vi "Examples - Basic ITC-SA.vi"(5 "Loop Controls":T7={"Heater"=FALSE, "Gas"=FALSE, "PID"=FALSE, "P (K)"=10.0, "I (mins)"=1.0, "D (mins)"=0.0, "Gas set point (%)"=0.0, "Htr Set V (V)"=0.0, "Target T(K)"=0.0, "Htr Set P (W)"=0.0, "Ramp Mode"=FALSE, "Target Rate(K/min)"=0.0, "Ramp End T(K)"=0.0} {"Ramp End T(K)" min=0.0 max=1000.0 step=0.0001 format="%_5g"; "Target Rate(K/min)" min=0.0 max=1000.0 step=0.0001 format="%_5g"; "Htr Set P (W)" min=0.0 max=80.0 step=0.0001 format="%_5g"; "Target T(K)" min=0.0 max=1000.0 step=0.0001 format="%_5g"; "Htr Set V (V)" min=0.0 max=40.0 step=0.0001 format="%_4g"; "Gas set point (%)" min=0.0 max=100.0 step=0.01 format="%_3g"; "D (mins)" min=0.0 max=300.0 step=0.001 format="%_4g"; "I (mins)" min=0.001 max=200.0 step=0.001 format="%_4g"; "P (K)" min=0.1 max=1000.0 step=0.001 format="%.3g"}, 11 "error in (no error)":errorcluster) -> (6 "Temperature (K)":dbl format="%_5g", 8 "Heater V (V)":dbl format="%_4g", 10 "Heater P (W)":dbl format="%_5g", 14 "Gas Open (%)":dbl(slide) scale=0.0..100.0, 15 "error out":errorcluster)   [LabVIEW 2013]
uses:
  <instrlib>/Mercury iXX/Public/Controls/Comms Transport Layer.ctl
  <instrlib>/Mercury iXX/Public/Controls/Serial Settings.ctl
  <instrlib>/Mercury iXX/Public/Controls/ISOBus Address.ctl
  <instrlib>/Mercury iXX/Public/Libraries/Control Loop/Controls/PID cluster.ctl
  <instrlib>/Mercury iXX/Public/Libraries/System/Open/Open System.vi
  <instrlib>/Mercury iXX/Public/Libraries/System/Read/Catalogue (Read).vi
  <instrlib>/Mercury iXX/Public/Libraries/Temperature/Open/Open Temperature Device.vi
  <instrlib>/Mercury iXX/Public/Libraries/Temperature/Configuration/Read/Nickname (Read).vi
  <instrlib>/Mercury iXX/Public/Libraries/Control Loop/Configuration/Read/Auto PID Filename (Read).vi
  <instrlib>/Mercury iXX/Public/Libraries/Control Loop/Configuration/Read/Heater Association (Read).vi
  <instrlib>/Mercury iXX/Public/Libraries/Heater/Open/Open Heater Device.vi
  <instrlib>/Mercury iXX/Public/Libraries/Heater/Configuration/Read/Voltage Limit (Read).vi
  <instrlib>/Mercury iXX/Public/Libraries/Control Loop/Configuration/Read/Auxiliary Association (Read).vi
  <instrlib>/Mercury iXX/Public/Libraries/Auxiliary/Open/Open Auxiliary Device.vi
  <instrlib>/Mercury iXX/Public/Libraries/Heater/Signals/Read/Voltage (Read).vi
  <instrlib>/Mercury iXX/Public/Libraries/Heater/Signals/Read/Power (Read).vi
  <instrlib>/Mercury iXX/Public/Libraries/Temperature/Signals/Read/Temperature (Read).vi
  <instrlib>/Mercury iXX/Public/Libraries/Control Loop/Configuration/Read/PID (Read).vi
  <instrlib>/Mercury iXX/Public/Libraries/Control Loop/Configuration/Read/PID Auto (Read).vi
  <instrlib>/Mercury iXX/Public/Libraries/Control Loop/Configuration/Read/Heater Auto (Read).vi
  <instrlib>/Mercury iXX/Public/Libraries/Control Loop/Configuration/Read/Flow Auto (Read).vi
  <instrlib>/Mercury iXX/Public/Libraries/Control Loop/Configuration/Read/Percentage Heat (Read).vi
  <instrlib>/Mercury iXX/Public/Libraries/Control Loop/Configuration/Set/Temperature Setpoint (Set).vi
  <instrlib>/Mercury iXX/Public/Libraries/Auxiliary/Signals/Read/Percent Open (Read).vi
  <instrlib>/Mercury iXX/Public/Libraries/Control Loop/Configuration/Set/Heater Auto (Set).vi
  <instrlib>/Mercury iXX/Public/Libraries/Control Loop/Configuration/Set/Flow Auto (Set).vi
  <instrlib>/Mercury iXX/Public/Libraries/Control Loop/Configuration/Set/PID Auto (Set).vi
  <instrlib>/Mercury iXX/Public/Libraries/Control Loop/Configuration/Set/D Value (Set).vi
  <instrlib>/Mercury iXX/Public/Libraries/Control Loop/Configuration/Set/I Value (Set).vi
  <instrlib>/Mercury iXX/Public/Libraries/Control Loop/Configuration/Set/P Value (Set).vi
  <instrlib>/Mercury iXX/Public/Libraries/Heater/Configuration/Read/Nominal Resistance (Read).vi
  <instrlib>/Mercury iXX/Public/Libraries/Control Loop/Configuration/Set/Percentage Heat (Set).vi
  <instrlib>/Mercury iXX/Public/Libraries/Control Loop/Configuration/Set/Percentage Flow (Set).vi
  <instrlib>/Mercury iXX/Mercury iXX.lvlib
  <instrlib>/Mercury iXX/Public/Libraries/System.lvlib
  <instrlib>/Mercury iXX/Public/Libraries/Temperature.lvlib
  <instrlib>/Mercury iXX/Public/Libraries/Heater.lvlib
  <instrlib>/Mercury iXX/Public/Libraries/Auxiliary.lvlib
  <instrlib>/Mercury iXX/Public/Libraries/Control Loop.lvlib
panel:
  in  "stop":bool
  in  "Tab Control":T1(tab)=enum."Configuration"
  in  "Connections":T5={"VISA resource name"="", "IP Address"="", "Comms Layer"=enum."Ethernet TCP/IP", "Serial Configuration"={"Baud Rate"=9600, "Parity"=0, "Data Bits"=8, "Stop Bits"=10, "Flow Control"=0}, "Clear Previous Connections (False)"=FALSE, "ID Query (True)"=TRUE, "ISOBUS address"=-1} {"Serial Configuration"."Flow Control" items=["None", "XON/XOFF", "RTS/CTS", "XON/XOFF & RTS/CTS", "DTR/DSR", "XON/XOFF & DTR/DSR"]; "Serial Configuration"."Stop Bits" items=["1.0"=10, "2.0"=20]; "Serial Configuration"."Data Bits" items=["7"=7, "8"=8]; "Serial Configuration"."Parity" items=["None", "Odd", "Even"]; "Serial Configuration"."Baud Rate" items=["300"=300, "600"=600, "1200"=1200, "2400"=2400, "4800"=4800, "9600"=9600, "19200"=19200]}
  out "# of Instruments":i32
  out "Serial Number(s)":string[](array[string])
  out "S/W Version(s)":string[](array[string])
  out "Devices":string[](array[string])
  in  "Connect":bool
  in  "Ramp mode: Interval between target updates (s)":dbl=10.0 min=0.25 max=60.0 step=0.25
  in  "Loop Dev Id's":T6={"Temperure Dev Id"="MB1.T1:TEMP", "Heater Dev Id"="MB0.H1:HTR", "Gas Cntl Dev Id"="DB4.G1:AUX", "Loop Has Gas Cntl?"=FALSE}
  out "Voltage Limit":dbl format="%.2g"
  out "Heater UID":string
  out "Gas Cntl UID":string
  out "Control Sensor":string
  out "Auto PID Filename:":string
  out "GAS":bool
  out "HEAT":bool
  out "Heater (%)":dbl(slide) scale=0.0..100.0
  out "String":string
  out "PID":T8 {"D" min=0.0 max=299.9 step=0.1 format="%#.1f"; "I" min=0.0 max=199.9 step=0.1 format="%#.1f"; "P" min=0.0 max=199.9 step=0.1 format="%#.1f"}
  out "PID":bool
  in  "Log file":string="C:\\temp\\test.lvm"
  out "Strip Chart":T9(graph)
  in  "Log?":bool
  # "Loop Mode\nAuto?"
  # "MercuryiTC-VI"
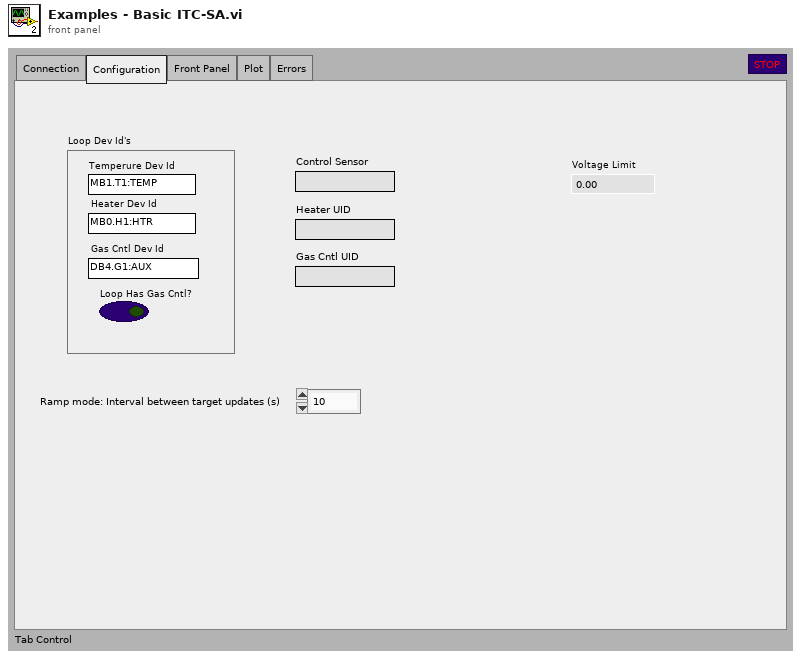
[diagram p1: front panel]
types:
  T1 = enum32{"Connection", "Configuration", "Front Panel", "Plot", "Errors"}
  T2 = typedef "Mercury iXX.lvlib/Comms Transport Layer.ctl" = enum16{"Ethernet TCP/IP", "USB", "ISOBus - RS-232", "GPIB"}
  T3 = typedef "Mercury iXX.lvlib/Serial Settings.ctl" = cluster{"Baud Rate":u32, "Parity":u16, "Data Bits":u16, "Stop Bits":u16, "Flow Control":u16}
  T4 = typedef "Mercury iXX.lvlib/ISOBus Address.ctl" = i32
  T5 = cluster{"VISA resource name":refnum<visa-resource-name>, "IP Address":string, "Comms Layer":T2, "Serial Configuration":T3, "Clear Previous Connections (False)":bool, "ID Query (True)":bool, "ISOBUS address":T4}
  T6 = cluster{"Temperure Dev Id":string, "Heater Dev Id":string, "Gas Cntl Dev Id":string, "Loop Has Gas Cntl?":bool}
  T7 = cluster{"Heater":bool, "Gas":bool, "PID":bool, "P (K)":dbl, "I (mins)":dbl, "D (mins)":dbl, "Gas set point (%)":dbl, "Htr Set V (V)":dbl, "Target T(K)":dbl, "Htr Set P (W)":dbl, "Ramp Mode":bool, "Target Rate(K/min)":dbl, "Ramp End T(K)":dbl}
  T8 = typedef "Mercury iXX.lvlib/Control Loop.lvlib/PID cluster.ctl" = cluster{"P":dbl, "I":dbl, "D":dbl}
  T9 = cluster{"Temperature":dbl, "Percentage Heat":dbl, "% Open":dbl}
  T10 = typedef "Mercury iXX.lvlib/Mercury Reference.ctl" = cluster{"Comms":refnum<visa-resource-name>, "Device ID":string[], "Comms Layer":T2, "Command":string, "Query reference":T11}
  T11 = typedef "Mercury iXX.lvlib/Query Dynamic Reference.ctl" = refnum<vi>
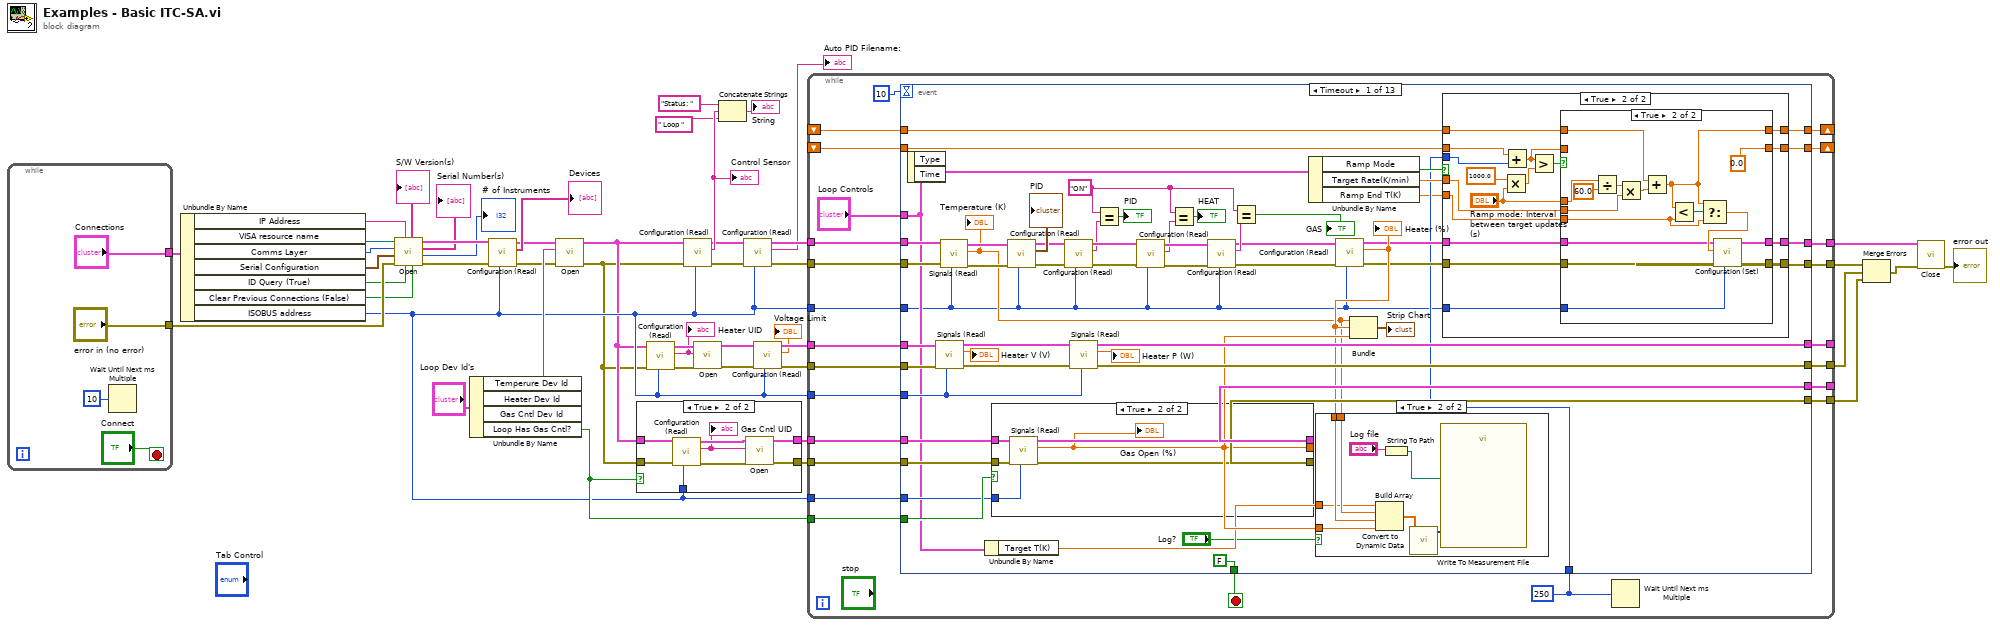
[diagram p0: block diagram]
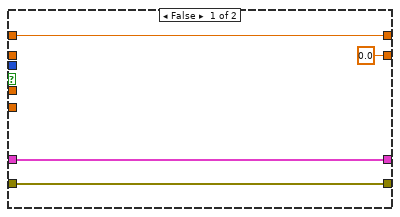
[diagram p3: hidden frame]
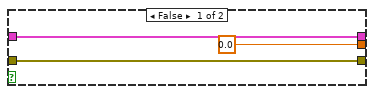
[diagram p6: hidden frame]
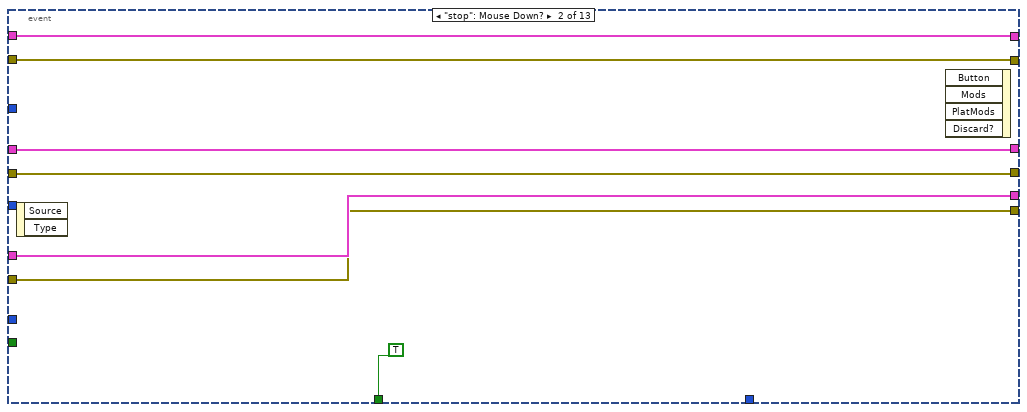
[diagram p7: hidden frame]
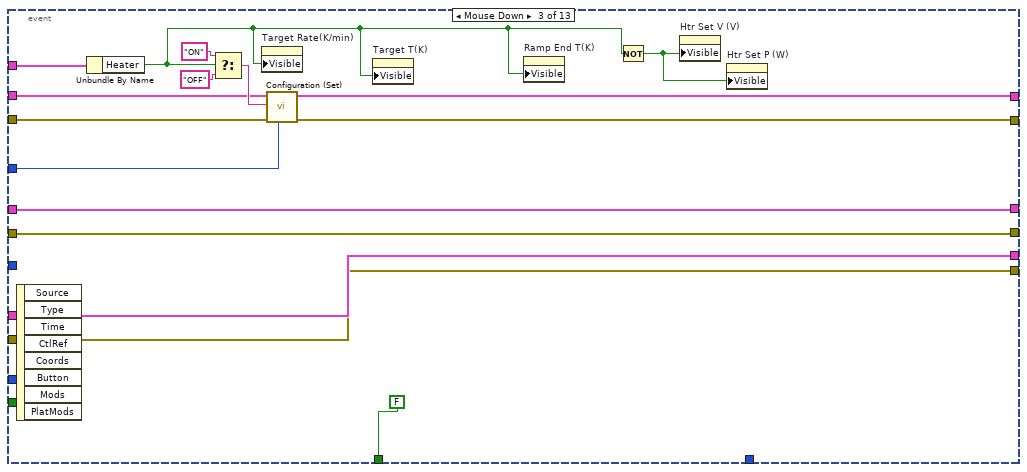
[diagram p8: hidden frame]
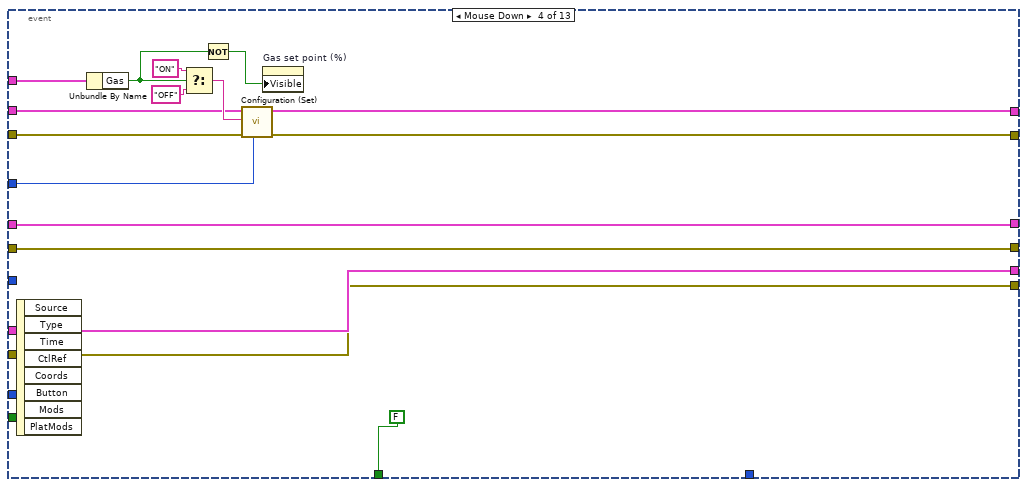
[diagram p9: hidden frame]
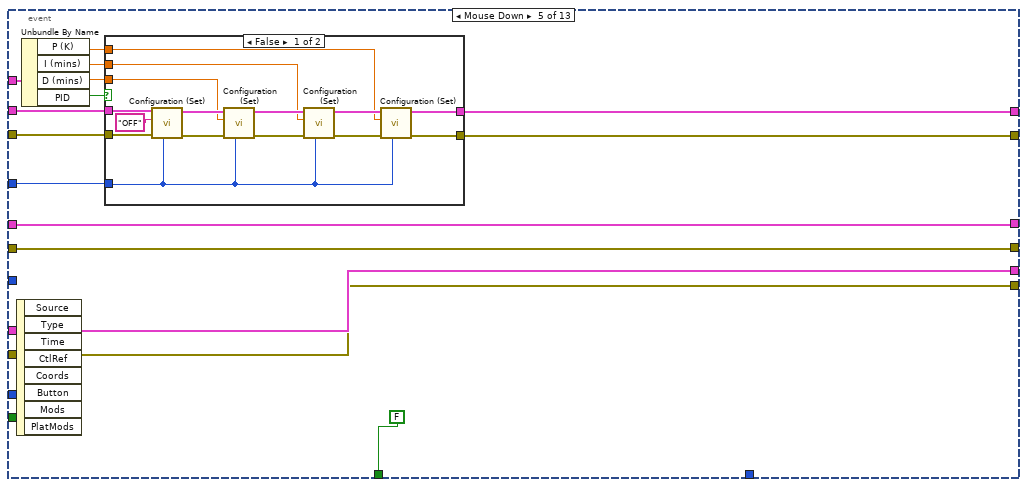
[diagram p10: hidden frame]
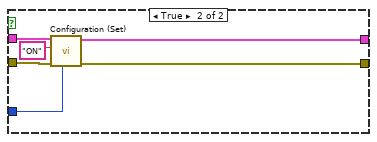
[diagram p11: hidden frame]
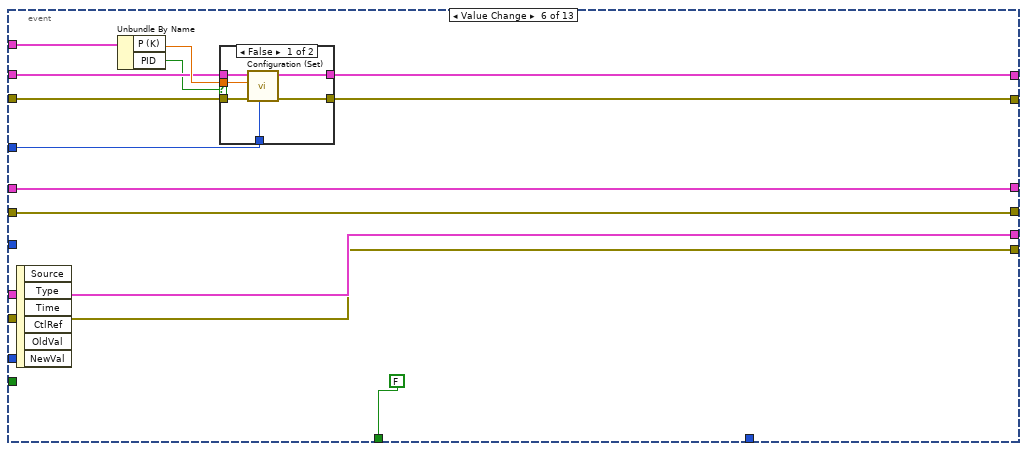
[diagram p12: hidden frame]
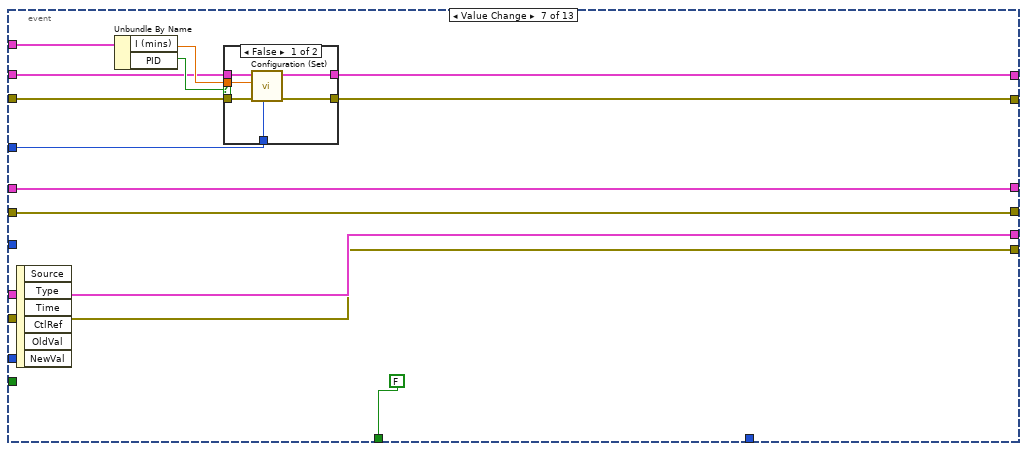
[diagram p14: hidden frame]
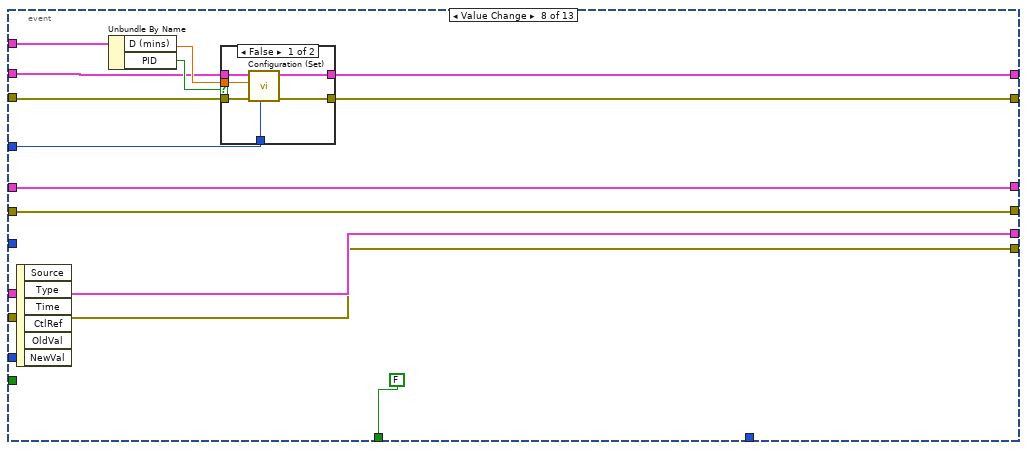
[diagram p16: hidden frame]
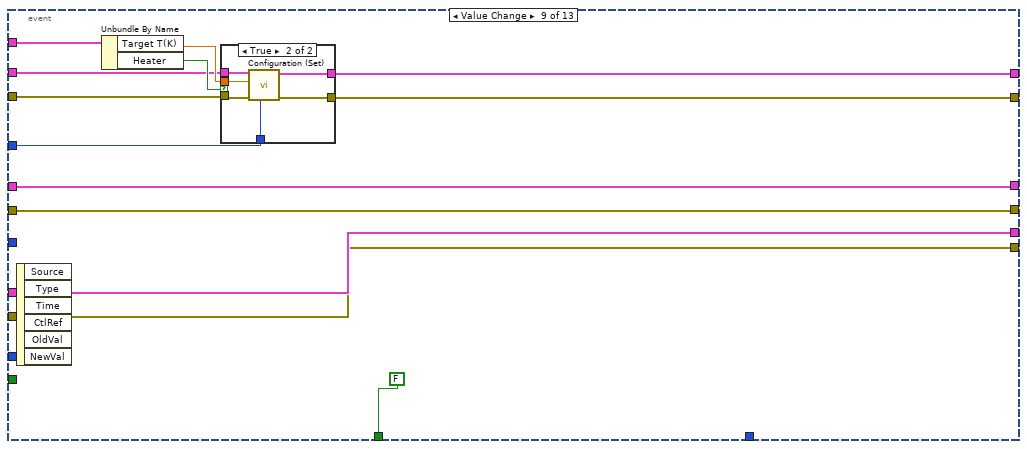
[diagram p18: hidden frame]
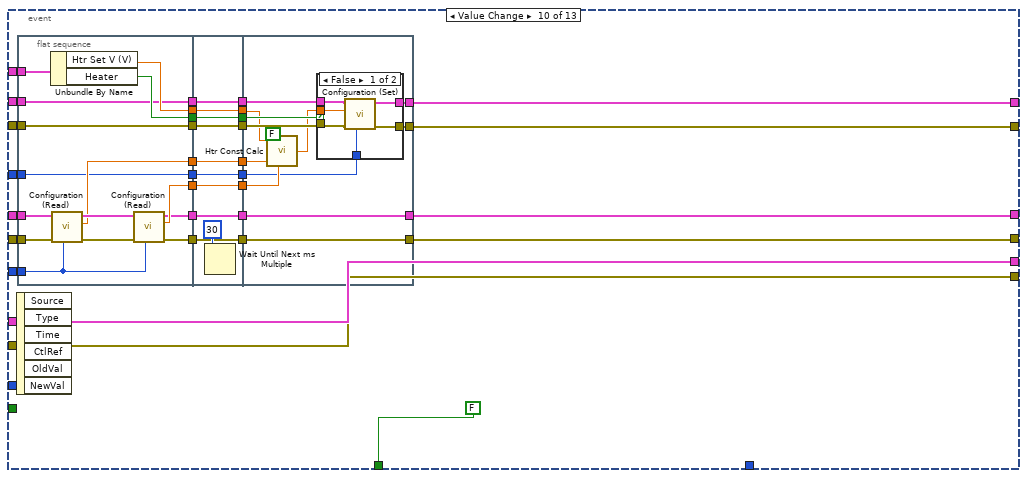
[diagram p20: hidden frame]
diagram:
  n1 = while {
    tunnel: ["error in (no error)"] -> w47
    tunnel: ["Connections"] -> w46
    stop <- "Connect" stop-if-true
    n2 = Wait Until Next ms Multiple(millisecond multiple=u32 10) -> ()  [unwired: 1 out]
  }
  n3 = Unbundle By Name(w46) -> ("IP Address"=w42:string, "VISA resource name"=w45:refnum<visa-resource-name>, "Comms Layer"=w44:T2, "Serial Configuration"=w43:T3, "ID Query (True)"=w41:bool, "Clear Previous Connections (False)"=w40:bool, "ISOBUS address"=w6:T4)
  n4 = call-poly <instrlib>:"Open.vi"("Clear Previous Connections (False)"=w40, "ID Query (True)"=w41, "IP Address"=w42, "error in (no error)"=w47, "Serial Configuration"=w43, "Comms Layer"=w44, "VISA resource name"=w45) -> ("error out"=w38:errorcluster, "# of Instruments"=→"# of Instruments":i32, "Serial Number(s)"=→"Serial Number(s)":string[], "Mercury Reference Out"=w39:T10, "S/W Version(s)"=→"S/W Version(s)":string[])
  n5 = Unbundle By Name("Loop Dev Id's") -> ("Temperure Dev Id"=w32:string, "Loop Has Gas Cntl?"=w29:bool)  [unwired: 2 out]
  n6 = call-poly <instrlib>:"Configuration (Read).vi"("ISOBUS address"=w6, "error in"=w38, "Mercury Reference In"=w39) -> ("error out"=w2:errorcluster, "Devices"=→"Devices":string[], "Mercury Reference Out"=w4:T10)  [unwired: 6 out]
  n7 = call-poly <instrlib>:"Open.vi"("error in (no error)"=w2, "Device Identifier"=w32, "Mercury Reference In"=w4) -> ("error out"=w1:errorcluster, "Mercury Reference Out"=w3:T10)  [unwired: 1 in, 6 out]
  n8 = case shown="True" w29 {
    tunnel: w3 -> [w53 w59]
    tunnel: w1 -> [w52 w58]
    tunnel: [w53 w61] -> w31
    tunnel: [w52 w60] -> w30
    tunnel: w6 -> [_ w55]
    frame False {
    }
    frame True {
      n9 = call-poly <instrlib>:"Configuration (Read).vi"("ISOBUS address"=w55, "error in"=w58, "Mercury Reference In"=w59) -> ("error out"=w56:errorcluster, "Auxiliary board UID"=w54:string, "Mercury Reference Out"=w57:T10)  [unwired: 6 out]
      "Gas Cntl UID" <- w54
      n10 = call-poly <instrlib>:"Open.vi"("error in (no error)"=w56, "Device Identifier"=w54, "Mercury Reference In"=w57) -> ("error out"=w60:errorcluster, "Mercury Reference Out"=w61:T10)  [unwired: 1 in, 6 out]
    }
  }
  n11 = call-poly <instrlib>:"Configuration (Read).vi"("ISOBUS address"=w6, "error in"=w1, "Mercury Reference In"=w3) -> ("error out"=w7:errorcluster, "Heater UID"=w5:string, "Mercury Reference Out"=w8:T10)  [unwired: 6 out]
  "Heater UID" <- w5
  n12 = call-poly <instrlib>:"Configuration (Read).vi"("ISOBUS address"=w6, "error in"=w1, "Mercury Reference In"=w3) -> ("error out"=w13:errorcluster, "Nickname"=w20:string, "Mercury Reference Out"=w14:T10)  [unwired: 6 out]
  "Control Sensor" <- w20
  n13 = call-poly <instrlib>:"Open.vi"("error in (no error)"=w7, "Device Identifier"=w5, "Mercury Reference In"=w8) -> ("error out"=w17:errorcluster, "Mercury Reference Out"=w18:T10)  [unwired: 7 out]
  n14 = Concatenate Strings("Status: ", w20, " Loop ") -> (→"String":string)
  n15 = call-poly <instrlib>:"Configuration (Read).vi"("ISOBUS address"=w6, "error in"=w13, "Mercury Reference In"=w14) -> ("error out"=w12:errorcluster, "Auto PID Filename"=→"Auto PID Filename:":string, "Mercury Reference Out"=w11:T10)  [unwired: 6 out]
  n16 = call-poly <instrlib>:"Configuration (Read).vi"("ISOBUS address"=w6, "error in"=w17, "Mercury Reference In"=w18) -> ("error out"=w15:errorcluster, "Voltage Limit"=→"Voltage Limit":dbl, "Mercury Reference Out"=w16:T10)  [unwired: 6 out]
  n17 = while {
    tunnel: w11 -> [w85]
    tunnel: w12 -> [w84]
    tunnel: w6 -> [w83]
    tunnel: w6 -> [w69]
    tunnel: w16 -> [w81]
    tunnel: w15 -> [w80]
    tunnel: w31 -> [w79]
    tunnel: w30 -> [w78]
    tunnel: w29 -> [w77]
    tunnel: [w76] -> w28
    tunnel: [w70] -> w26
    tunnel: [w75] -> _
    tunnel: [w74] -> w25
    tunnel: [w73] -> _
    tunnel: [w72] -> w24
    tunnel: w6 -> [w67]
    shift-right: [w65] -> _
    shift-left: _ -> [w64]
    shift-right: [w63] -> _
    shift-left: _ -> [w62]
    stop <- w82 stop-if-true
    w66 = u32 250 ("millisecond multiple")
    n18 = event shown="[0] Timeout" {
      selector: _ -> [_ _ _ _ _ _ _ _ _ _ _ _ _]
      dyn-events: _ -> [_ _ _ _ _ _ _ _ _ _ _ _ _]
      timeout: 10 -> [_ _ _ _ _ _ _ _ _ _ _ _ _]
      tunnel: w85 -> [w141 w205 w219 w235 w245 w285 w305 w326 w347 w374 w455 w524 w541]
      tunnel: w84 -> [w140 w204 w218 w234 w246 w284 w304 w325 w348 w381 w452 w523 w540]
      tunnel: w83 -> [w91 _ w217 w233 w247 w283 w301 w322 w344 w369 w449 w522 w539]
      tunnel: [FALSE TRUE FALSE FALSE FALSE FALSE FALSE FALSE FALSE FALSE FALSE FALSE _] -> w82
      tunnel: w69 -> [w127 _ _ _ _ _ _ _ _ _ _ _ _]
      tunnel: w81 -> [w138 w203 w213 w230 w253 w279 w300 w320 w343 w390 w459 w519 _]
      tunnel: w80 -> [w137 w202 w212 w229 w252 w278 w299 w319 w342 w389 w458 w518 _]
      tunnel: w79 -> [w136 w201 w211 w228 w251 w277 w298 w318 w341 w368 w445 w517 _]
      tunnel: w78 -> [w135 w200 w210 w227 w250 w276 w297 w317 w340 w367 w446 w516 _]
      tunnel: w77 -> [w134 _ _ _ _ _ _ _ _ _ _ _ _]
      tunnel: [w96 w205 w216 w232 w240 w282 w303 w324 w346 w366 w444 w521 w537] -> w76
      tunnel: [w126 w203 w213 w230 w253 w279 w300 w320 w343 w364 w442 w519 _] -> w75
      tunnel: [w125 w202 w212 w229 w252 w278 w299 w319 w342 w361 w439 w518 _] -> w74
      tunnel: [w131 w201 w211 w228 w251 w277 w298 w318 w341 w368 w445 w517 _] -> w73
      tunnel: [w130 w200 w210 w227 w250 w276 w297 w317 w340 w367 w446 w516 _] -> w72
      tunnel: "Loop Controls" -> [w99 _ w209 w225 w248 w286 w306 w328 w338 w388 w460 w525 _]
      tunnel: [w95 w204 w215 w231 w239 w281 w302 w323 w345 w365 w443 w520 w536] -> w70
      tunnel: w67 -> [w123 _ _ _ _ _ _ _ _ w372 w448 _ _]
      tunnel: w66 -> [w92 _ _ _ _ _ _ _ _ _ _ _ _]
      tunnel: [w89 _ _ _ _ _ _ _ _ _ _ _ _] -> w65
      tunnel: w64 -> [w88 _ _ _ _ _ _ _ _ _ _ _ _]
      tunnel: [w86 _ _ _ _ _ _ _ _ _ _ _ w538] -> w63
      tunnel: w62 -> [w87 _ _ _ _ _ _ _ _ _ _ _ _]
      event Timeout {
        w111 = "ON"
        n19 = event-data() -> ()  [unwired: 3 out]
        n20 = call-poly <instrlib>:"Signals (Read).vi"("ISOBUS address"=w123, "error in"=w137, "Mercury Reference In"=w138) -> ("error out"=w128:errorcluster, "Voltage"=→"Heater V (V)":dbl, "Mercury Reference Out"=w129:T10)  [unwired: 6 out]
        n21 = call-poly <instrlib>:"Signals (Read).vi"("ISOBUS address"=w91, "error in"=w140, "Mercury Reference In"=w141) -> ("error out"=w132:errorcluster, "Temperature"=w102:dbl, "Mercury Reference Out"=w133:T10)  [unwired: 6 out]
        "Temperature (K)" <- w102
        n22 = Unbundle By Name(w99) -> ("Target T(K)"=w101:dbl)
        n23 = case shown="True" w134 {
          tunnel: w127 -> [_ w199]
          tunnel: w136 -> [w192 w198]
          tunnel: w135 -> [w193 w197]
          tunnel: [w192 w196] -> w131
          tunnel: [w193 w195] -> w130
          tunnel: [0.0 ("% Open") w194] -> w104
          frame False {
          }
          frame True {
            n24 = call-poly <instrlib>:"Signals (Read).vi"("ISOBUS address"=w199, "error in"=w197, "Mercury Reference In"=w198) -> ("error out"=w195:errorcluster, "% Open"=w194:dbl, "Mercury Reference Out"=w196:T10)  [unwired: 6 out]
            "Gas Open (%)" <- w194
          }
        }
        n25 = call-poly <instrlib>:"Configuration (Read).vi"("ISOBUS address"=w91, "error in"=w132, "Mercury Reference In"=w133) -> ("error out"=w117:errorcluster, "PID"=→"PID":T8, "Mercury Reference Out"=w120:T10)  [unwired: 6 out]
        n26 = call-poly <instrlib>:"Configuration (Read).vi"("ISOBUS address"=w91, "error in"=w117, "Mercury Reference In"=w120) -> ("error out"=w116:errorcluster, "PID Auto"=w114:string, "Mercury Reference Out"=w119:T10)  [unwired: 6 out]
        n27 = call-poly <instrlib>:"Signals (Read).vi"("ISOBUS address"=w123, "error in"=w128, "Mercury Reference In"=w129) -> ("error out"=w125:errorcluster, "Power"=→"Heater P (W)":dbl, "Mercury Reference Out"=w126:T10)  [unwired: 6 out]
        n28 = Equal?(x=w111, y=w114) -> (x = y?=→"PID":bool)
        n29 = call-poly <instrlib>:"Configuration (Read).vi"("ISOBUS address"=w91, "error in"=w116, "Mercury Reference In"=w119) -> ("error out"=w115:errorcluster, "Heater Auto"=w112:string, "Mercury Reference Out"=w118:T10)  [unwired: 6 out]
        n30 = Equal?(x=w111, y=w112) -> (x = y?=→"HEAT":bool)
        n31 = call-poly <instrlib>:"Configuration (Read).vi"("ISOBUS address"=w91, "error in"=w115, "Mercury Reference In"=w118) -> ("error out"=w106:errorcluster, "Flow Auto"=w110:string, "Mercury Reference Out"=w107:T10)  [unwired: 6 out]
        n32 = Equal?(x=w111, y=w110) -> (x = y?=→"GAS":bool)
        n33 = Unbundle By Name(w99) -> ("Ramp Mode"=w94:bool, "Target Rate(K/min)"=w93:dbl, "Ramp End T(K)"=w90:dbl)
        n34 = call-poly <instrlib>:"Configuration (Read).vi"("ISOBUS address"=w91, "error in"=w106, "Mercury Reference In"=w107) -> ("error out"=w97:errorcluster, "Percentage Heat"=w103:dbl, "Mercury Reference Out"=w98:T10)  [unwired: 6 out]
        "Heater (%)" <- w103
        n35 = case shown="True" "Log?" {
          tunnel: w104 -> [_ w190]
          tunnel: w103 -> [_ w189]
          tunnel: w102 -> [_ w188]
          tunnel: w101 -> [_ w187]
          frame False {
          }
          frame True {
            n36 = Build Array(w187, w188, w189, w190) -> (w186:dbl[])
            n37 = String To Path(string="Log file") -> (path=w183:path)
            n38 = call "Convert to Dynamic Data"("Array"=w186) -> ("Dynamic Data Type"=w185:dynamicdata)  [unwired: 3 in]
            n39 = call "Write To Measurement File"("Signals"=w185, "Filename"=w183) -> ()  [unwired: 15 in, 3 out]
          }
        }
        n40 = Bundle("Temperature"=w102, "Percentage Heat"=w103, "% Open"=w104) -> (→"Strip Chart":T9)  [unwired: 1 out]
        n41 = case shown="True" w94 {
          tunnel: w98 -> [w145 w149]
          tunnel: w97 -> [w144 w150]
          tunnel: [w145 w157] -> w96
          tunnel: [w144 w156] -> w95
          tunnel: w93 -> [_ w152]
          tunnel: w92 -> [_ w162]
          tunnel: w91 -> [_ w155]
          tunnel: w90 -> [_ w151]
          tunnel: [0.0 ("f") w159] -> w89
          tunnel: w88 -> [_ w158]
          tunnel: w87 -> [w142 w147]
          tunnel: [w142 w146] -> w86
          frame False {
          }
          frame True {
            n42 = Multiply(x=1000.0 ("y"), y="Ramp mode: Interval between target updates (s)") -> (x*y=w161:dbl)
            n43 = Add(x=w158, y=w162) -> (x+y=w148:dbl)
            n44 = Greater?(x=w148, y=w161) -> (0:w160:bool)
            n45 = case shown="True" w160 {
              tunnel: [w164 0.0 ("f")] -> w159
              tunnel: w149 -> [w166 w168]
              tunnel: w150 -> [w165 w167]
              tunnel: [w166 w181] -> w157
              tunnel: [w165 w180] -> w156
              tunnel: w155 -> [_ w179]
              tunnel: "Ramp mode: Interval between target updates (s)" -> [_ w177]
              tunnel: w152 -> [_ w175]
              tunnel: w151 -> [_ w173]
              tunnel: w148 -> [w164 _]
              tunnel: w147 -> [w163 w171]
              tunnel: [w163 w169] -> w146
              frame False {
              }
              frame True {
                n46 = Divide(x=w177, y=60.0) -> (x/y=w176:dbl)
                n47 = Multiply(x=w176, y=w175) -> (x*y=w170:dbl)
                n48 = Add(x=w171, y=w170) -> (x+y=w169:dbl)
                n49 = Less?(x=w169, y=w173) -> (x < y?=w174:bool)
                n50 = Select(t=w169, s=w174, f=w173) -> (s? t:f=w172:dbl)
                n51 = call-poly <instrlib>:"Configuration (Set).vi"("ISOBUS address"=w179, "error in"=w167, "Temperature setpoint"=w172, "Mercury Reference In"=w168) -> ("error out"=w180:errorcluster, "Mercury Reference Out"=w181:T10)  [unwired: 1 in, 5 out]
              }
            }
          }
        }
      }
      event "stop": Mouse Down? {
        n52 = event-data() -> ()  [unwired: 3 out]
        n53 = event-data() -> ()  [unwired: 1 in, 5 out]
      }
      event "Loop Controls.Heater": Mouse Down {
        n54 = event-data() -> ()  [unwired: 9 out]
        n55 = Unbundle By Name(w209) -> ("Heater"=w207:bool)
        n56 = Select(t="ON", s=w207, f="OFF") -> (s? t:f=w220:string)
        n57 = property on="Target Rate(K/min)" class="DigNum (strict)"("Visible"=w207) -> ()  [unwired: 2 in, 2 out]
        n58 = call-poly <instrlib>:"Configuration (Set).vi"("ISOBUS address"=w217, "error in"=w218, "Heater Auto"=w220, "Mercury Reference In"=w219) -> ("error out"=w215:errorcluster, "Mercury Reference Out"=w216:T10)  [unwired: 6 out]
        n59 = property on="Target T(K)" class="DigNum (strict)"("Visible"=w207) -> ()  [unwired: 2 in, 2 out]
        n60 = property on="Ramp End T(K)" class="DigNum (strict)"("Visible"=w207) -> ()  [unwired: 2 in, 2 out]
        n61 = Not(x=w207) -> (.not. x?=w208:bool)
        n62 = property on="Htr Set V (V)" class="DigNum (strict)"("Visible"=w208) -> ()  [unwired: 2 in, 2 out]
        n63 = property on="Htr Set P (W)" class="DigNum (strict)"("Visible"=w208) -> ()  [unwired: 2 in, 2 out]
      }
      event "Loop Controls.Gas": Mouse Down {
        n64 = event-data() -> ()  [unwired: 9 out]
        n65 = Unbundle By Name(w225) -> ("Gas"=w224:bool)
        n66 = Select(t="ON", s=w224, f="OFF") -> (s? t:f=w236:string)
        n67 = Not(x=w224) -> (.not. x?=w223:bool)
        n68 = call-poly <instrlib>:"Configuration (Set).vi"("ISOBUS address"=w233, "error in"=w234, "Flow Auto"=w236, "Mercury Reference In"=w235) -> ("error out"=w231:errorcluster, "Mercury Reference Out"=w232:T10)  [unwired: 6 out]
        n69 = property on="Gas set point (%)" class="DigNum (strict)"("Visible"=w223) -> ()  [unwired: 2 in, 2 out]
      }
      event "Loop Controls.PID": Mouse Down {
        n70 = event-data() -> ()  [unwired: 9 out]
        n71 = Unbundle By Name(w248) -> ("P (K)"=w241:dbl, "I (mins)"=w242:dbl, "D (mins)"=w243:dbl, "PID"=w244:bool)
        n72 = case shown="False" w244 {
          tunnel: w247 -> [w257 w274]
          tunnel: w246 -> [w267 w273]
          tunnel: w245 -> [w268 w272]
          tunnel: [w262 w270] -> w240
          tunnel: [w258 w269] -> w239
          tunnel: w243 -> [w256 _]
          tunnel: w242 -> [w255 _]
          tunnel: w241 -> [w254 _]
          frame False {
            n73 = call-poly <instrlib>:"Configuration (Set).vi"("ISOBUS address"=w257, "error in"=w267, "PID Auto"="OFF", "Mercury Reference In"=w268) -> ("error out"=w261:errorcluster, "Mercury Reference Out"=w265:T10)  [unwired: 6 out]
            n74 = call-poly <instrlib>:"Configuration (Set).vi"("ISOBUS address"=w257, "error in"=w261, "D Value"=w256, "Mercury Reference In"=w265) -> ("error out"=w260:errorcluster, "Mercury Reference Out"=w264:T10)  [unwired: 1 in, 5 out]
            n75 = call-poly <instrlib>:"Configuration (Set).vi"("ISOBUS address"=w257, "error in"=w260, "I Value"=w255, "Mercury Reference In"=w264) -> ("error out"=w259:errorcluster, "Mercury Reference Out"=w263:T10)  [unwired: 1 in, 5 out]
            n76 = call-poly <instrlib>:"Configuration (Set).vi"("ISOBUS address"=w257, "error in"=w259, "P Value"=w254, "Mercury Reference In"=w263) -> ("error out"=w258:errorcluster, "Mercury Reference Out"=w262:T10)  [unwired: 1 in, 5 out]
          }
          frame True {
            n77 = call-poly <instrlib>:"Configuration (Set).vi"("ISOBUS address"=w274, "error in"=w273, "PID Auto"="ON", "Mercury Reference In"=w272) -> ("error out"=w269:errorcluster, "Mercury Reference Out"=w270:T10)  [unwired: 6 out]
          }
        }
      }
      event "Loop Controls.P (K)": Value Change {
        n78 = event-data() -> ()  [unwired: 7 out]
        n79 = Unbundle By Name(w286) -> ("P (K)"=w287:dbl, "PID"=w280:bool)
        n80 = case shown="False" w280 {
          tunnel: w287 -> [w293 _]
          tunnel: w285 -> [w292 w295]
          tunnel: w284 -> [w291 w294]
          tunnel: w283 -> [w290 _]
          tunnel: [w289 w295] -> w282
          tunnel: [w288 w294] -> w281
          frame False {
            n81 = call-poly <instrlib>:"Configuration (Set).vi"("ISOBUS address"=w290, "error in"=w291, "P Value"=w293, "Mercury Reference In"=w292) -> ("error out"=w288:errorcluster, "Mercury Reference Out"=w289:T10)  [unwired: 1 in, 5 out]
          }
          frame True {
          }
        }
      }
      event "Loop Controls.I (mins)": Value Change {
        n82 = event-data() -> ()  [unwired: 7 out]
        n83 = Unbundle By Name(w306) -> ("I (mins)"=w308:dbl, "PID"=w307:bool)
        n84 = case shown="False" w307 {
          tunnel: w308 -> [w309 _]
          tunnel: [w314 w316] -> w303
          tunnel: [w313 w315] -> w302
          tunnel: w305 -> [w312 w316]
          tunnel: w304 -> [w311 w315]
          tunnel: w301 -> [w310 _]
          frame False {
            n85 = call-poly <instrlib>:"Configuration (Set).vi"("ISOBUS address"=w310, "error in"=w311, "I Value"=w309, "Mercury Reference In"=w312) -> ("error out"=w313:errorcluster, "Mercury Reference Out"=w314:T10)  [unwired: 1 in, 5 out]
          }
          frame True {
          }
        }
      }
      event "Loop Controls.D (mins)": Value Change {
        n86 = event-data() -> ()  [unwired: 7 out]
        n87 = Unbundle By Name(w328) -> ("D (mins)"=w329:dbl, "PID"=w327:bool)
        n88 = case shown="False" w327 {
          tunnel: w329 -> [w331 _]
          tunnel: [w335 w337] -> w324
          tunnel: [w334 w336] -> w323
          tunnel: w326 -> [w333 w337]
          tunnel: w325 -> [w332 w336]
          tunnel: w322 -> [w330 _]
          frame False {
            n89 = call-poly <instrlib>:"Configuration (Set).vi"("ISOBUS address"=w330, "error in"=w332, "D Value"=w331, "Mercury Reference In"=w333) -> ("error out"=w334:errorcluster, "Mercury Reference Out"=w335:T10)  [unwired: 1 in, 5 out]
          }
          frame True {
          }
        }
      }
      event "Loop Controls.Target T(K)": Value Change {
        n90 = event-data() -> ()  [unwired: 7 out]
        n91 = Unbundle By Name(w338) -> ("Target T(K)"=w350:dbl, "Heater"=w349:bool)
        n92 = case shown="True" w349 {
          tunnel: w350 -> [_ w355]
          tunnel: [w352 w358] -> w346
          tunnel: [w351 w357] -> w345
          tunnel: w348 -> [w351 w356]
          tunnel: w347 -> [w352 w354]
          tunnel: w344 -> [_ w353]
          frame False {
          }
          frame True {
            n93 = call-poly <instrlib>:"Configuration (Set).vi"("ISOBUS address"=w353, "error in"=w356, "Temperature setpoint"=w355, "Mercury Reference In"=w354) -> ("error out"=w357:errorcluster, "Mercury Reference Out"=w358:T10)  [unwired: 1 in, 5 out]
          }
        }
      }
      event "Loop Controls.Htr Set V (V)": Value Change {
        n94 = event-data() -> ()  [unwired: 7 out]
        n95 = flat-sequence {
          tunnel: w390 -> [w403]
          tunnel: w389 -> [w402]
          tunnel: w388 -> [w399]
          tunnel: [w405] -> w387
          tunnel: [w404] -> w386
          tunnel: [w398] -> w382
          tunnel: w381 -> [w398]
          tunnel: [w397] -> w380
          tunnel: [w396] -> w378
          tunnel: [w395] -> w375
          tunnel: w374 -> [w395]
          tunnel: w372 -> [w394]
          tunnel: [w393] -> w370
          tunnel: w369 -> [w393]
          tunnel: [w392] -> w362
          tunnel: [w391] -> w359
          tunnel: w387 -> [w415]
          tunnel: w386 -> [w414]
          tunnel: [w415] -> w385
          tunnel: [w414] -> w384
          tunnel: [w413] -> w383
          tunnel: w382 -> [w413]
          tunnel: w380 -> [w411]
          tunnel: [w411] -> w379
          tunnel: w378 -> [w410]
          tunnel: [w410] -> w377
          tunnel: [w409] -> w376
          tunnel: w375 -> [w409]
          tunnel: [w408] -> w371
          tunnel: w370 -> [w408]
          tunnel: [w407] -> w363
          tunnel: w362 -> [w407]
          tunnel: [w406] -> w360
          tunnel: w359 -> [w406]
          tunnel: w385 -> [w426]
          tunnel: w384 -> [w428]
          tunnel: w383 -> [w427]
          tunnel: w379 -> [w425]
          tunnel: w377 -> [w424]
          tunnel: w376 -> [w421]
          tunnel: [w420] -> w366
          tunnel: [w419] -> w365
          tunnel: w371 -> [w418]
          tunnel: [w417] -> w364
          tunnel: w363 -> [w417]
          tunnel: [w416] -> w361
          tunnel: w360 -> [w416]
          frame #0 {
            n96 = Unbundle By Name(w399) -> ("Htr Set V (V)"=w405:dbl, "Heater"=w404:bool)
            n97 = call-poly <instrlib>:"Configuration (Read).vi"("ISOBUS address"=w394, "error in"=w402, "Mercury Reference In"=w403) -> ("error out"=w400:errorcluster, "Voltage Limit"=w397:dbl, "Mercury Reference Out"=w401:T10)  [unwired: 6 out]
            n98 = call-poly <instrlib>:"Configuration (Read).vi"("ISOBUS address"=w394, "error in"=w400, "Mercury Reference In"=w401) -> ("error out"=w391:errorcluster, "Nominal Resistance"=w396:dbl, "Mercury Reference Out"=w392:T10)  [unwired: 6 out]
          }
          frame #1 {
            n99 = Wait Until Next ms Multiple(millisecond multiple=u32 30) -> ()  [unwired: 1 out]
          }
          frame #2 {
            n100 = call <instrlib>:"Htr Const Calc.vi"("Htr Set V (V)"=w426, "Htr Const Mode"=FALSE, "Htr V_Lim (V)"=w425, "Htr Res (ohms)"=w424) -> ("Htr Set (%)"=w422:dbl)  [unwired: 1 in]
            n101 = case shown="False" w428 {
              tunnel: [w434 w436] -> w420
              tunnel: [w433 w435] -> w419
              tunnel: w427 -> [w432 w435]
              tunnel: w422 -> [w430 _]
              tunnel: w421 -> [w431 w436]
              tunnel: w418 -> [w429 _]
              frame False {
                n102 = call-poly <instrlib>:"Configuration (Set).vi"("ISOBUS address"=w429, "error in"=w432, "Percentage Heat"=w430, "Mercury Reference In"=w431) -> ("error out"=w433:errorcluster, "Mercury Reference Out"=w434:T10)  [unwired: 1 in, 5 out]
              }
              frame True {
              }
            }
          }
        }
      }
      event "Heater P (W)": Value Change {
        n103 = event-data() -> ()  [unwired: 7 out]
        n104 = flat-sequence {
          tunnel: [w483] -> w468
          tunnel: [w482] -> w467
          tunnel: [w479] -> w466
          tunnel: [w478] -> w465
          tunnel: w460 -> [w477]
          tunnel: w459 -> [w476]
          tunnel: w458 -> [w475]
          tunnel: [w474] -> w456
          tunnel: w455 -> [w474]
          tunnel: [w473] -> w453
          tunnel: w452 -> [w473]
          tunnel: [w472] -> w450
          tunnel: w449 -> [w472]
          tunnel: w448 -> [w471]
          tunnel: [w470] -> w440
          tunnel: [w469] -> w437
          tunnel: w468 -> [w493]
          tunnel: w467 -> [w492]
          tunnel: [w493] -> w464
          tunnel: [w492] -> w463
          tunnel: w466 -> [w490]
          tunnel: [w490] -> w462
          tunnel: w465 -> [w489]
          tunnel: [w489] -> w461
          tunnel: [w488] -> w457
          tunnel: w456 -> [w488]
          tunnel: [w487] -> w454
          tunnel: w453 -> [w487]
          tunnel: [w486] -> w451
          tunnel: w450 -> [w486]
          tunnel: [w485] -> w441
          tunnel: w440 -> [w485]
          tunnel: [w484] -> w438
          tunnel: w437 -> [w484]
          tunnel: w464 -> [w499]
          tunnel: w463 -> [w506]
          tunnel: w462 -> [w505]
          tunnel: w461 -> [w504]
          tunnel: [w501] -> w444
          tunnel: [w500] -> w443
          tunnel: w457 -> [w498]
          tunnel: w454 -> [w497]
          tunnel: w451 -> [w496]
          tunnel: [w495] -> w442
          tunnel: w441 -> [w495]
          tunnel: [w494] -> w439
          tunnel: w438 -> [w494]
          frame #0 {
            n105 = Unbundle By Name(w477) -> ("Htr Set P (W)"=w483:dbl, "Heater"=w482:bool)
            n106 = call-poly <instrlib>:"Configuration (Read).vi"("ISOBUS address"=w471, "error in"=w475, "Mercury Reference In"=w476) -> ("error out"=w480:errorcluster, "Voltage Limit"=w479:dbl, "Mercury Reference Out"=w481:T10)  [unwired: 6 out]
            n107 = call-poly <instrlib>:"Configuration (Read).vi"("ISOBUS address"=w471, "error in"=w480, "Mercury Reference In"=w481) -> ("error out"=w469:errorcluster, "Nominal Resistance"=w478:dbl, "Mercury Reference Out"=w470:T10)  [unwired: 6 out]
          }
          frame #1 {
            n108 = Wait Until Next ms Multiple(millisecond multiple=u32 30) -> ()  [unwired: 1 out]
          }
          frame #2 {
            n109 = call <instrlib>:"Htr Const Calc.vi"("Htr Const Mode"=TRUE, "Htr Set P (W)"=w499, "Htr V_Lim (V)"=w505, "Htr Res (ohms)"=w504) -> ("Htr Set (%)"=w502:dbl)  [unwired: 1 in]
            n110 = case shown="False" w506 {
              tunnel: [w512 w514] -> w501
              tunnel: [w511 w513] -> w500
              tunnel: w502 -> [w510 _]
              tunnel: w498 -> [w509 w514]
              tunnel: w497 -> [w508 w513]
              tunnel: w496 -> [w507 _]
              frame False {
                n111 = call-poly <instrlib>:"Configuration (Set).vi"("ISOBUS address"=w507, "error in"=w508, "Percentage Heat"=w510, "Mercury Reference In"=w509) -> ("error out"=w511:errorcluster, "Mercury Reference Out"=w512:T10)  [unwired: 1 in, 5 out]
              }
              frame True {
              }
            }
          }
        }
      }
      event "Loop Controls.Gas set point (%)": Value Change {
        n112 = event-data() -> ()  [unwired: 7 out]
        n113 = Unbundle By Name(w525) -> ("Gas set point (%)"=w527:dbl, "Gas"=w526:bool)
        n114 = case shown="False" w526 {
          tunnel: w527 -> [w530 _]
          tunnel: [w533 w535] -> w521
          tunnel: [w532 w534] -> w520
          tunnel: w524 -> [w531 w535]
          tunnel: w523 -> [w529 w534]
          tunnel: w522 -> [w528 _]
          frame False {
            n115 = call-poly <instrlib>:"Configuration (Set).vi"("ISOBUS address"=w528, "error in"=w529, "Percentage Flow"=w530, "Mercury Reference In"=w531) -> ("error out"=w532:errorcluster, "Mercury Reference Out"=w533:T10)  [unwired: 1 in, 5 out]
          }
          frame True {
          }
        }
      }
      event "Loop Controls.Ramp Mode": Value Change {
        n116 = event-data() -> ()  [unwired: 7 out]
        n117 = call-poly <instrlib>:"Signals (Read).vi"("ISOBUS address"=w539, "error in"=w540, "Mercury Reference In"=w541) -> ("error out"=w536:errorcluster, "Temperature"=w538:dbl, "Mercury Reference Out"=w537:T10)  [unwired: 6 out]
      }
    }
    n118 = Wait Until Next ms Multiple(millisecond multiple=w66) -> ()  [unwired: 1 out]
  }
  n119 = Merge Errors(w26, w25, w24) -> (w27:errorcluster)
  n120 = call <instrlib>:"Close.vi"("error in (no error)"=w27, "Mercury Reference"=w28) -> ("error out"=→"error out":errorcluster)  [unwired: 9 out]
